vi "HEWH Assemble HEWH Diagnostics Data.vi"(0 "Input Updated Data (No GEA) 2":string[][](array[string])=[["APPLIANCE SOFTWARE VERSION (0x0100)", ""], ["USER SET MODE (0X4020)", ""], ["OPERATING MODE (0X4021)", ""], ["USER SETPOINT (0x4024)", ""], ["ACTUAL SETPOINT (0x4026)", ""], ["MODEL DESIGNATOR (0x4042)", ""], ["DLB RELAY (0x4068)", ""], ["COMPRESSOR RELAY (0x4068)", ""], ["LOWER ELEMENT RELAY (0x4068)", ""], ["UPPER ELEMENT RELAY (0x4068)", ""], ["FAN (0x4068)", ""], ["T1 TEMP (0x405F)", ""], ["T2 TEMP (0x4060)", ""], ["T3A TEMP (0x4061)", ""], ["T3B TEMP (0x4062)", ""], ["T4 TEMP (0x4063)", ""], ["T5 TEMP (0x4064)", ""], ["VOLTAGE (0x4066)", ""], ["DLB CURRENT (0x4065)", ""], ["EEV POSITION (0x4067)", ""], ["FLOW EVENTS (0x4069)", ""], ["STORED THERMAL CAPACITANCE (0x4058)", ""], ["AVAILABLE THERMAL CAPACITANCE (0x4059)", ""], ["MAXIMUM THERMAL CAPACITANCE (0X405A)", ""], ["VOLTAGE PULSES (0X404F)", ""], ["TANK SIZE (0X4041)", ""]], 5 "UE":i16, 7 "LE":i16, 11 "Error In":errorcluster, 12 "Comp":i16, 13 "Fan":i16, 14 "DLB":i16) -> (4 "Output Updated Data (No GEA)":string[][](array[string]), 15 "Error Out":errorcluster)   [LabVIEW 2016]
uses:
  Utility/GEA2 Commands/HEWH/Type Definitions/GEA2 Commands WaterHeater GEA2 Data.ctl
  Utility/GEA2 Commands/HEWH/Type Definitions/GEA2 Commands Button Status.ctl
  Utility/GEA2 Commands/HEWH/Type Definitions/GEA2 Commands Status Query.ctl
  Utility/GEA2 Commands/HEWH/Type Definitions/GEA2 Commands Service Error Codes.ctl
panel:
  in  "Header":string[](array[string])
  in  "Water Heater GEA2 Data in":T1 {"Hyperterminal Data"."CRC" format="%x"; "Hyperterminal Data"."Length" format="%x"; "Hyperterminal Data"."Command" format="%x"; "Hyperterminal Data"."Destination" format="%x"; "Hyperterminal Data"."Source" format="%x"}
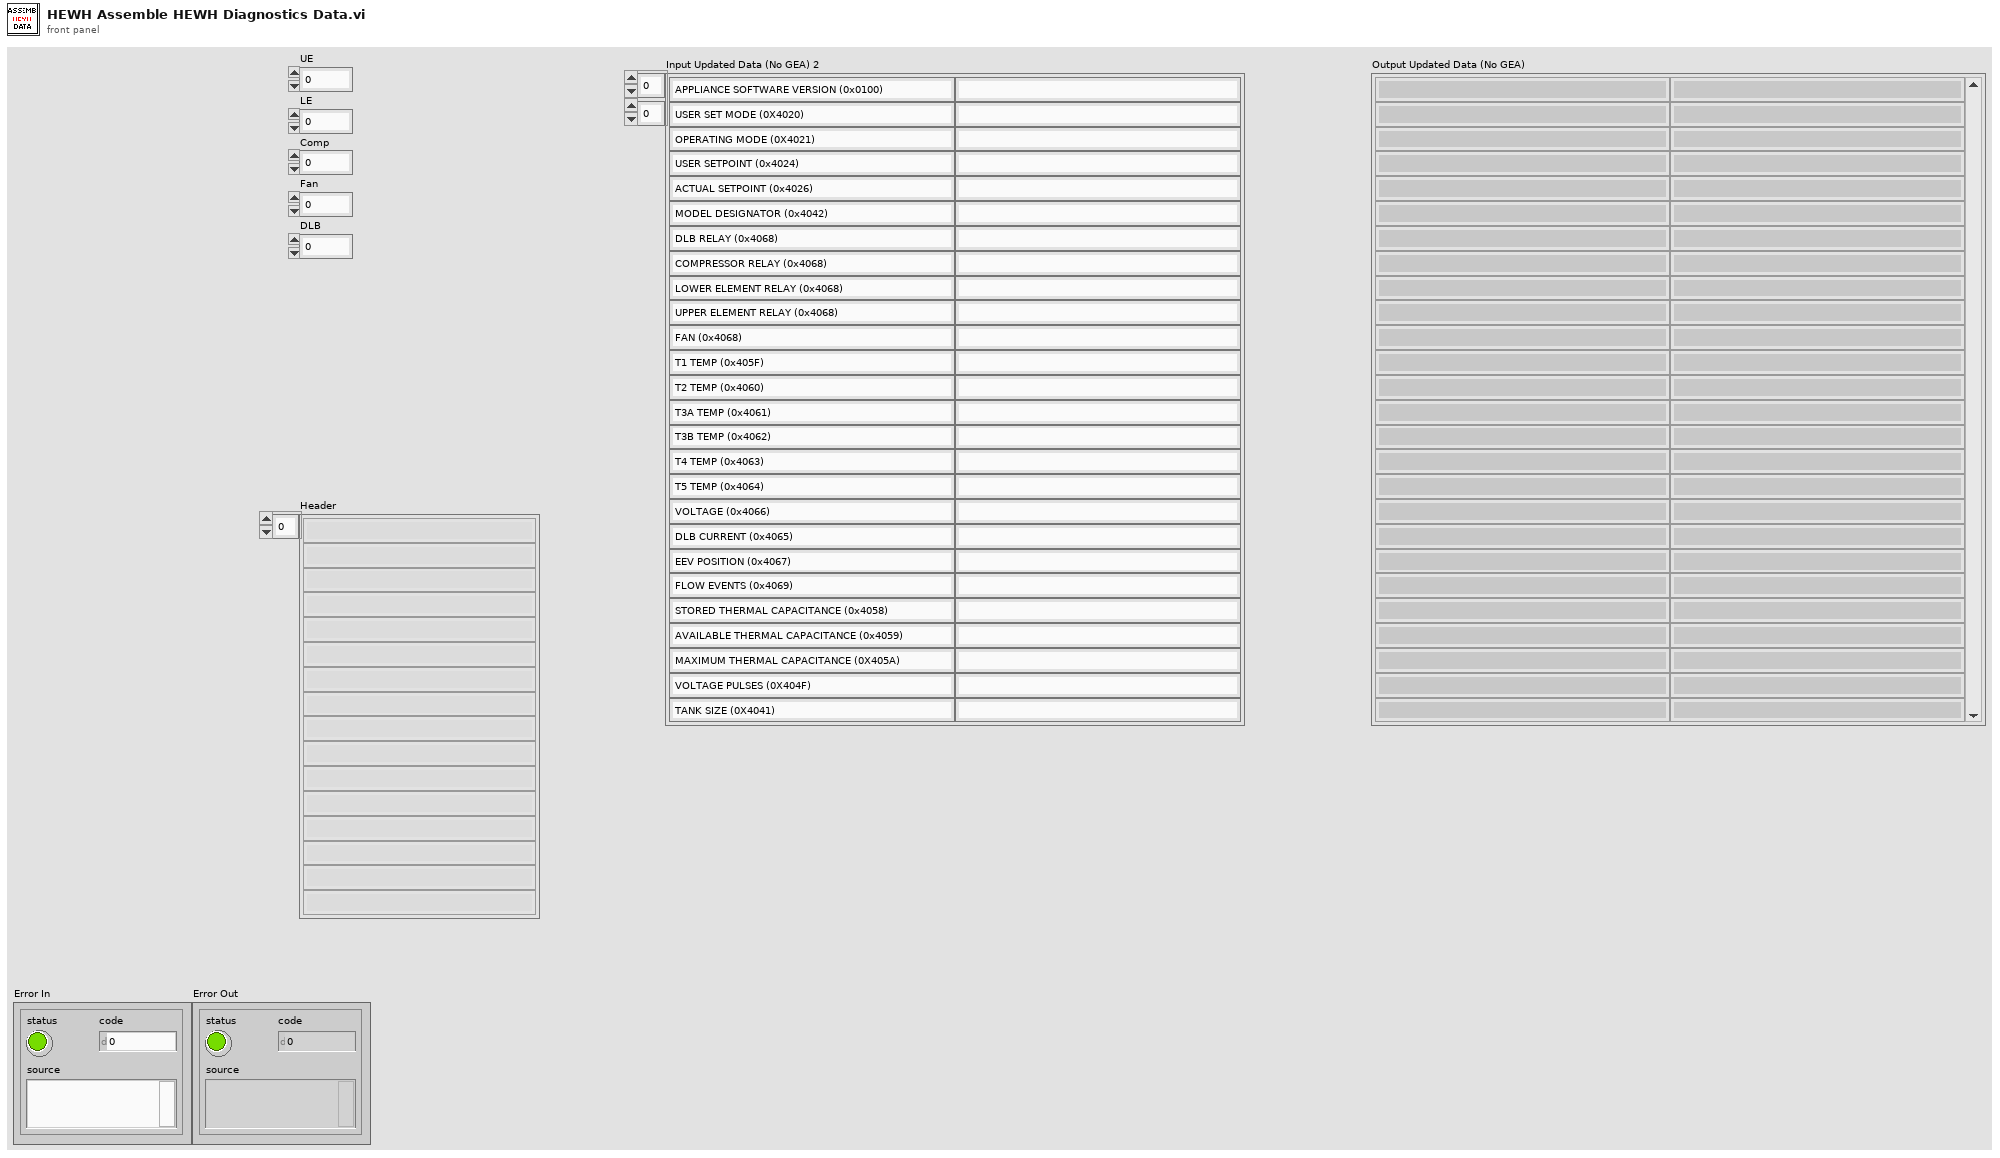
[diagram p1: front panel]
types:
  T1 = typedef "GEA2 Commands WaterHeater GEA2 Data.ctl" = cluster{"GEA2 Label Array":string[], "PID_PARAMETERS":string[][], "SUPPORTED_MODES":string[][], "Button Status":T2, "Status Query":T3, "Service Error Codes":T4, "HEM_KWH_DATA":string[][], "OTHER_FAULT_COUNTS":string[][], "GEA2 Raw Message":string, "Hyperterminal Data":cluster{"Source":u8, "Destination":u8, "Command":u8, "Length":u8, "CRC":u16, "UE - state (1/0 on off)":u8, "LE - state (1/0 on off)":u8, "Comp - state (1/0 on off)":u8, "Fan  - state (1/0 on off)":u8, "Setpoint Deg F":i32, "T2(TankSensor)":dbl, "T3A(EvapIn)":dbl, "T3B(EvapOut)":dbl, "T4(CompressorDischarge)":dbl, "T5(Ambient)":dbl, "Current":dbl, "Voltage (Volts)":u16, "EEV Position (0-480)":u16, "Reason for last heating cycle termination":u16, "Reason Data word 1":string, "Reason Data word 2":string, "Reason Data word 3":string, "Reason Data word 4":string, "SW Debug Data":string, "Flow Events (Bit Encoded)":u16, "Heating Control Mode":u16}, "Extra Data":cluster{"Water Capacity (Gallons)":u32, "Max Vacation Duration Days":u32, "Min Vacation Duration Days":u32, "Max Set Point (Deg F)":u32, "Min Set Point (Deg F)":u32, "T5 Resistance":u32, "T4 Resistance":u32, "T3B Resistance":u32, "T2 Resistance":u32, "STD_ELEC_RANGE":string, "SS_FAULT_COUNTS":string, "SERIAL_NUMBER":string, "READ_PERSONALITY":u8, "RQST_OVERRIDE_STATUS":string, "MODEL_SELECT_AD_VALUE":u32, "MODEL NUMBER":string, "IDLB_RESISTANCE":u32, "DSM Override Status":string, "RQST_DATA_FROM_Memory":string, "RQST_DATA_FROM_DATA_FLASH":string, "RQST_CURRENT_PID_SH_TARGET":u16, "Unit System Mode":string}}
  T2 = typedef "GEA2 Commands Button Status.ctl" = cluster{"Switch 1":bool, "Switch 2":bool, "Switch 3":bool, "Switch 4":bool, "Switch 5":bool, "Switch 6":bool, "Switch 7":bool, "Switch 8":bool, "Switch 9":bool, "Switch 10":bool, "Switch 11":bool, "Switch 12":bool, "Switch 13":bool, "Switch 14":bool, "Switch 15":bool, "Switch 16":bool}
  T3 = typedef "GEA2 Commands Status Query.ctl" = cluster{"Days Remaining (For Std Electric and Vacation)":u8, "Unit Status":string, "Current Tank Temp in Deg F":u8, "Current Setpoint in Deg F":u8, "Filter Status (% used)":u8, "Fallback Status (Fallback heating mode)":string, "Fallback Temp":u8, "\"Set Mode\" Selection":string}
  T4 = typedef "GEA2 Commands Service Error Codes.ctl" = cluster{"Reserved":bool, "Reserved 1":bool, "Reserved 2":bool, "Reserved 3":bool, "Reserved 4":bool, "Reserved 5":bool, "Reserved 6":bool, "Reserved 7":bool, "DataFlash Fail Status":bool, "Stuck Key Fail Status":bool, "Dry Tank Fail Status":bool, "Miswire Fail Status":bool, "Reserved 8":bool, "Reserved 9":bool, "Reserved 10":bool, "Reserved 11":bool, "UE Fail Status":bool, "LE Fail Status":bool, "Filter Fail Status":bool, "T3A Fail Status":bool, "T3B Fail Status":bool, "T4 Fail Status":bool, "T5 Fail Status":bool, "T2 Fail Status":bool, "SS Cond A Status":bool, "SS Cond B Status":bool, "SS Cond C Status":bool, "SS Cond D Status":bool, "SS Cond E Status":bool, "SS Cond F Status":bool, "SS Fan Status":bool, "CMP Fail Status":bool}
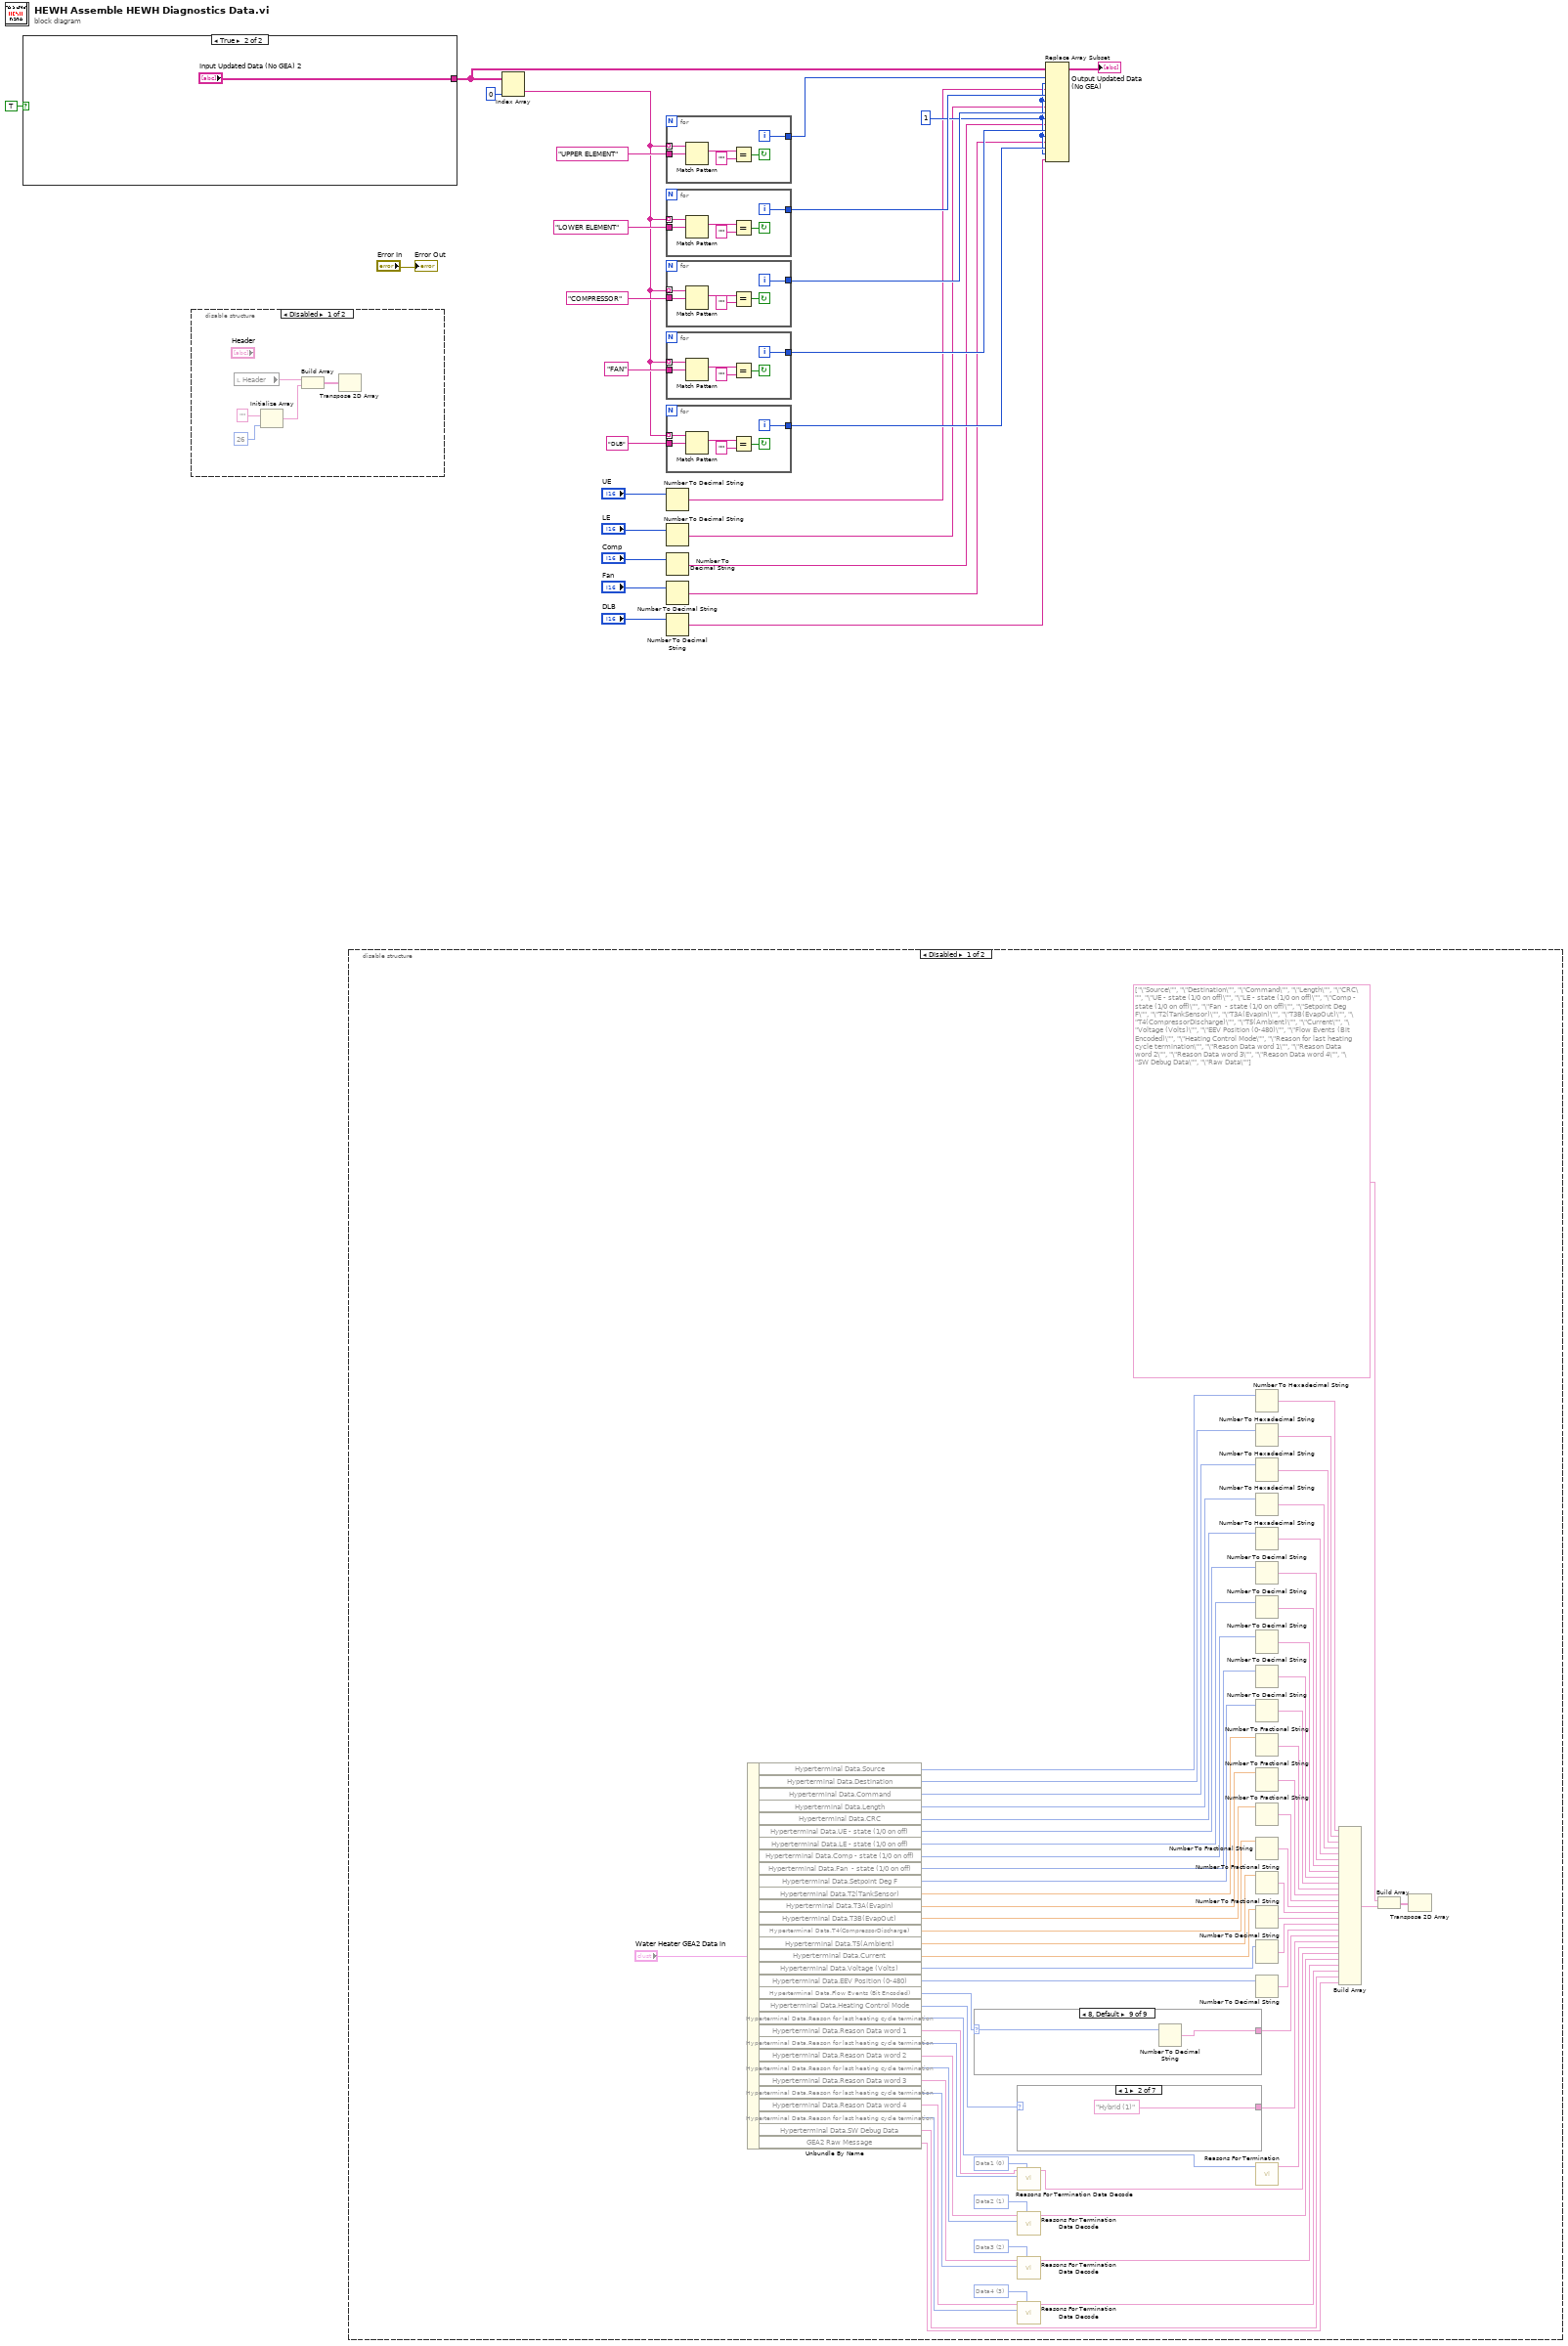
[diagram p0: block diagram]
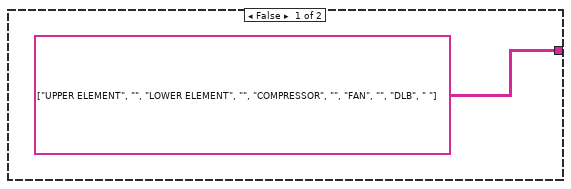
[diagram p2: hidden frame]
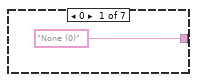
[diagram p4: hidden frame]
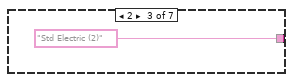
[diagram p5: hidden frame]
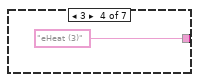
[diagram p6: hidden frame]
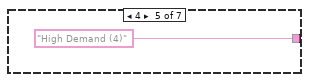
[diagram p7: hidden frame]
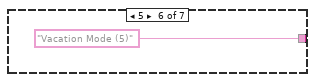
[diagram p8: hidden frame]
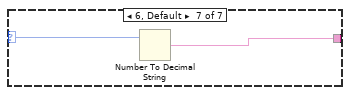
[diagram p9: hidden frame]
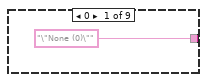
[diagram p10: hidden frame]
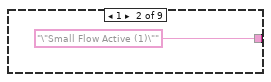
[diagram p11: hidden frame]
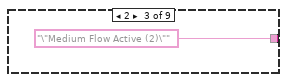
[diagram p12: hidden frame]
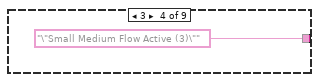
[diagram p13: hidden frame]
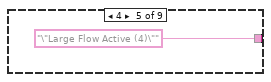
[diagram p14: hidden frame]
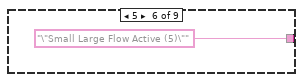
[diagram p15: hidden frame]
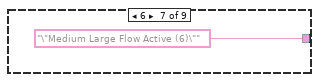
[diagram p16: hidden frame]
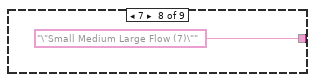
[diagram p17: hidden frame]
diagram:
  w8 = 1 ("disabled index (col)")
  n1 = case shown="True" TRUE {
    tunnel: [string[][] [["UPPER ELEMENT", ""], ["LOWER ELEMENT", ""], ["COMPRESSOR", ""], ["FAN", ""], ["DLB", " "]] ("ERD Data") "Input Updated Data (No GEA) 2"] -> w21
    frame False {
    }
    frame True {
    }
  }
  n2 = disable-structure shown="Disabled" {
    frame Disabled {
      n3 = local read "Header"() -> (w34:string[])
      n4 = Initialize Array("", 26 ("dimension size")) -> (w31:string[])
      n5 = Build Array(w34, w31) -> (w30:string[][])
      n6 = Transpose 2D Array(2D array=w30) -> ()  [unwired: 1 out]
    }
    frame Enabled {
    }
  }
  n7 = disable-structure shown="Disabled" {
    frame Disabled {
      w56 = u16 3 items=["Data1", "Data2", "Data3", "Data4"] ("Data")
      w55 = u16 2 items=["Data1", "Data2", "Data3", "Data4"] ("Data")
      w54 = u16 1 items=["Data1", "Data2", "Data3", "Data4"] ("Data")
      w53 = u16 0 items=["Data1", "Data2", "Data3", "Data4"] ("Data")
      n8 = Unbundle By Name("Water Heater GEA2 Data in") -> ("Hyperterminal Data.Source"=w35:u8, "Hyperterminal Data.Destination"=w36:u8, "Hyperterminal Data.Command"=w37:u8, "Hyperterminal Data.Length"=w38:u8, "Hyperterminal Data.CRC"=w39:u16, "Hyperterminal Data.UE - state (1/0 on off)"=w40:u8, "Hyperterminal Data.LE - state (1/0 on off)"=w41:u8, "Hyperterminal Data.Comp - state (1/0 on off)"=w42:u8, "Hyperterminal Data.Fan  - state (1/0 on off)"=w43:u8, "Hyperterminal Data.Setpoint Deg F"=w44:i32, "Hyperterminal Data.T2(TankSensor)"=w45:dbl, "Hyperterminal Data.T3A(EvapIn)"=w46:dbl, "Hyperterminal Data.T3B(EvapOut)"=w47:dbl, "Hyperterminal Data.T4(CompressorDischarge)"=w48:dbl, "Hyperterminal Data.T5(Ambient)"=w49:dbl, "Hyperterminal Data.Current"=w50:dbl, "Hyperterminal Data.Voltage (Volts)"=w51:u16, "Hyperterminal Data.EEV Position (0-480)"=w52:u16, "Hyperterminal Data.Flow Events (Bit Encoded)"=w81:u16, "Hyperterminal Data.Heating Control Mode"=w93:u16, "Hyperterminal Data.Reason for last heating cycle termination"=w86:u16, "Hyperterminal Data.Reason Data word 1"=w95:string, "Hyperterminal Data.Reason for last heating cycle termination"=w87:u16, "Hyperterminal Data.Reason Data word 2"=w96:string, "Hyperterminal Data.Reason for last heating cycle termination"=w88:u16, "Hyperterminal Data.Reason Data word 3"=w97:string, "Hyperterminal Data.Reason for last heating cycle termination"=w89:u16, "Hyperterminal Data.Reason Data word 4"=w98:string, "Hyperterminal Data.Reason for last heating cycle termination"=w90:u16, "Hyperterminal Data.SW Debug Data"=w80:string, "GEA2 Raw Message"=w82:string)
      n9 = case shown="8, Default" w81 {
        selector: w81 -> [_ _ _ _ _ _ _ _ w116]
        tunnel: ["\"None (0)\"" "\"Small Flow Active (1)\"" "\"Medium Flow Active (2)\"" "\"Small Medium Flow Active (3)\"" "\"Large Flow Active (4)\"" "\"Small Large Flow Active (5)\"" "\"Medium Large Flow Active (6)\"" "\"Small Medium Large Flow (7)\"" w115] -> w92
        frame 0 {
        }
        frame 1 {
        }
        frame 2 {
        }
        frame 3 {
        }
        frame 4 {
        }
        frame 5 {
        }
        frame 6 {
        }
        frame 7 {
        }
        frame 8, Default {
          n10 = Number To Decimal String(number=w116) -> (decimal integer string=w115:string)  [unwired: 1 in]
        }
      }
      n11 = case shown="1" w93 {
        selector: w93 -> [_ _ _ _ _ _ w106]
        tunnel: ["None (0)" "Hybrid (1)" "Std Electric (2)" "eHeat (3)" "High Demand (4)" "Vacation Mode (5)" w105] -> w94
        frame 0 {
        }
        frame 1 {
        }
        frame 2 {
        }
        frame 3 {
        }
        frame 4 {
        }
        frame 5 {
        }
        frame 6, Default {
          n12 = Number To Decimal String(number=w106) -> (decimal integer string=w105:string)  [unwired: 1 in]
        }
      }
      n13 = call "Reasons For Termination Data Decode.vi"("Data"=w53, "Reason for Last Heating Cycle Termination"=w87, "Reason Data Word"=w95) -> ("Reason Data Word 1 Output"=w76:string)  [unwired: 8 in]
      n14 = call "Reasons For Termination Data Decode.vi"("Data"=w54, "Reason for Last Heating Cycle Termination"=w88, "Reason Data Word"=w96) -> ("Reason Data Word 1 Output"=w77:string)  [unwired: 8 in]
      n15 = call "Reasons For Termination Data Decode.vi"("Data"=w55, "Reason for Last Heating Cycle Termination"=w89, "Reason Data Word"=w97) -> ("Reason Data Word 1 Output"=w78:string)  [unwired: 8 in]
      n16 = call "Reasons For Termination Data Decode.vi"("Data"=w56, "Reason for Last Heating Cycle Termination"=w90, "Reason Data Word"=w98) -> ("Reason Data Word 1 Output"=w79:string)  [unwired: 8 in]
      n17 = Number To Hexadecimal String(2:w35) -> (0:w57:string)  [unwired: 1 in]
      n18 = Number To Hexadecimal String(2:w36) -> (0:w58:string)  [unwired: 1 in]
      n19 = Number To Hexadecimal String(2:w37) -> (0:w59:string)  [unwired: 1 in]
      n20 = Number To Hexadecimal String(2:w38) -> (0:w60:string)  [unwired: 1 in]
      n21 = Number To Hexadecimal String(2:w39) -> (0:w61:string)  [unwired: 1 in]
      n22 = Number To Decimal String(number=w40) -> (decimal integer string=w62:string)  [unwired: 1 in]
      n23 = Number To Decimal String(number=w41) -> (decimal integer string=w63:string)  [unwired: 1 in]
      n24 = Number To Decimal String(number=w42) -> (decimal integer string=w64:string)  [unwired: 1 in]
      n25 = Number To Decimal String(number=w43) -> (decimal integer string=w65:string)  [unwired: 1 in]
      n26 = Number To Decimal String(number=w44) -> (decimal integer string=w66:string)  [unwired: 1 in]
      n27 = Number To Fractional String(number=w45) -> (F-format string=w67:string)  [unwired: 3 in]
      n28 = Number To Fractional String(number=w46) -> (F-format string=w68:string)  [unwired: 3 in]
      n29 = Number To Fractional String(number=w47) -> (F-format string=w69:string)  [unwired: 3 in]
      n30 = Number To Fractional String(number=w48) -> (F-format string=w70:string)  [unwired: 3 in]
      n31 = Number To Fractional String(number=w49) -> (F-format string=w71:string)  [unwired: 3 in]
      n32 = Number To Fractional String(number=w50) -> (F-format string=w72:string)  [unwired: 3 in]
      n33 = Number To Decimal String(number=w51) -> (decimal integer string=w73:string)  [unwired: 1 in]
      n34 = Number To Decimal String(number=w52) -> (decimal integer string=w74:string)  [unwired: 1 in]
      n35 = call "Reasons For Termination.vi"("Reason for last heating cycle termination"=w86) -> ("String"=w75:string)  [unwired: 10 in]
      n36 = Build Array(w57, w58, w59, w60, w61, w62, w63, w64, w65, w66, w67, w68, w69, w70, w71, w72, w73, w74, w92, w94, w75, w76, w77, w78, w79, w80, w82) -> (w83:string[])
      n37 = Build Array(string[] ["\"Source\"", "\"Destination\"", "\"Command\"", "\"Length\"", "\"CRC\"", "\"UE - state (1/0 on off)\"", "\"LE - state (1/0 on off)\"", "\"Comp - state (1/0 on off)\"", "\"Fan  - state (1/0 on off)\"", "\"Setpoint Deg F\"", "\"T2(TankSensor)\"", "\"T3A(EvapIn)\"", "\"T3B(EvapOut)\"", "\"T4(CompressorDischarge)\"", "\"T5(Ambient)\"", "\"Current\"", "\"Voltage (Volts)\"", "\"EEV Position (0-480)\"", "\"Flow Events (Bit Encoded)\"", "\"Heating Control Mode\"", "\"Reason for last heating cycle termination\"", "\"Reason Data word 1\"", "\"Reason Data word 2\"", "\"Reason Data word 3\"", "\"Reason Data word 4\"", "\"SW Debug Data\"", "\"Raw Data\""] ("GEA2 Label Array"), w83) -> (w85:string[][])
      n38 = Transpose 2D Array(2D array=w85) -> ()  [unwired: 1 out]
    }
    frame Enabled {
    }
  }
  n39 = Index Array(array=w21, index (col)=0 ("disabled index (col)")) -> (element=w14:string[])  [unwired: 1 in]
  n40 = for {
    tunnel: w14 -> [w122] mode=indexing
    tunnel: "UPPER ELEMENT" -> [w121]
    tunnel: [w120] -> w13
    i -> [w120]
    stop <- w117 continue-if-true
    n41 = Match Pattern(string=w122, regular expression=w121) -> (match substring=w119:string)  [unwired: 1 in, 3 out]
    n42 = Equal?(x=w119, y="") -> (x = y?=w117:bool)
  }
  n43 = for {
    tunnel: w14 -> [w128] mode=indexing
    tunnel: "LOWER ELEMENT" -> [w127]
    tunnel: [w126] -> w12
    i -> [w126]
    stop <- w123 continue-if-true
    n44 = Match Pattern(string=w128, regular expression=w127) -> (match substring=w125:string)  [unwired: 1 in, 3 out]
    n45 = Equal?(x=w125, y="") -> (x = y?=w123:bool)
  }
  n46 = for {
    tunnel: w14 -> [w134] mode=indexing
    tunnel: "COMPRESSOR" -> [w133]
    tunnel: [w132] -> w11
    i -> [w132]
    stop <- w129 continue-if-true
    n47 = Match Pattern(string=w134, regular expression=w133) -> (match substring=w131:string)  [unwired: 1 in, 3 out]
    n48 = Equal?(x=w131, y="") -> (x = y?=w129:bool)
  }
  n49 = for {
    tunnel: w14 -> [w140] mode=indexing
    tunnel: "FAN" -> [w139]
    tunnel: [w138] -> w10
    i -> [w138]
    stop <- w135 continue-if-true
    n50 = Match Pattern(string=w140, regular expression=w139) -> (match substring=w137:string)  [unwired: 1 in, 3 out]
    n51 = Equal?(x=w137, y="") -> (x = y?=w135:bool)
  }
  n52 = for {
    tunnel: w14 -> [w146] mode=indexing
    tunnel: "DLB" -> [w145]
    tunnel: [w144] -> w9
    i -> [w144]
    stop <- w141 continue-if-true
    n53 = Match Pattern(string=w146, regular expression=w145) -> (match substring=w143:string)  [unwired: 1 in, 3 out]
    n54 = Equal?(x=w143, y="") -> (x = y?=w141:bool)
  }
  n55 = Number To Decimal String(number="UE") -> (decimal integer string=w7:string)  [unwired: 1 in]
  n56 = Number To Decimal String(number="LE") -> (decimal integer string=w6:string)  [unwired: 1 in]
  n57 = Number To Decimal String(number="Comp") -> (decimal integer string=w5:string)  [unwired: 1 in]
  n58 = Number To Decimal String(number="Fan") -> (decimal integer string=w4:string)  [unwired: 1 in]
  n59 = Number To Decimal String(number="DLB") -> (decimal integer string=w3:string)  [unwired: 1 in]
  n60 = Replace Array Subset(array=w21, new element #1=w7, index (row) #1=w13, index (col) #1=w8, new element #2=w6, index (row) #2=w12, index (col) #2=w8, new element #3=w5, index (row) #3=w11, index (col) #3=w8, new element #4=w4, index (row) #4=w10, index (col) #4=w8, new element #5=w3, index (row) #5=w9, index (col) #5=w8) -> (→"Output Updated Data (No GEA)":string[][])
  "Error Out" <- "Error In"
